vi "ATSpectrograph_getEvent_reportedFilterPosition.vi"(8 "error in (no error)":errorcluster, 11 "logevent_reportedFilterPosition_Ctl":T1) -> (0 "error out":errorcluster, 2 "function return":i32, 3 "logevent_reportedFilterPosition_Ctl out":T1)   [LabVIEW 2016, in "SALLV_ATSpectrograph.lvlib"]
doc: "int ATSpectrograph_shm_getEvent_reportedFilterPositionLV(ATSpectrograph_logevent_reportedFilterPositionLV *logevent_reportedFilterPosition_Ctl );"
uses:
  SALLV_ATSpectrograph.lvlib
  DataTypes/logevent_reportedFilterPosition.ctl
  SALLV_ATSpectrograph.so
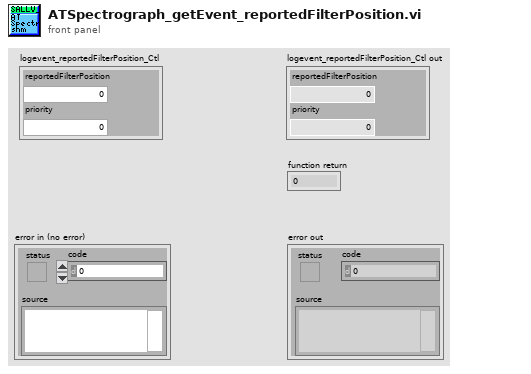
[diagram p1: front panel]
types:
  T1 = typedef "SALLV_ATSpectrograph.lvlib/logevent_reportedFilterPosition.ctl" = cluster{"reportedFilterPosition":i32, "priority":i32}
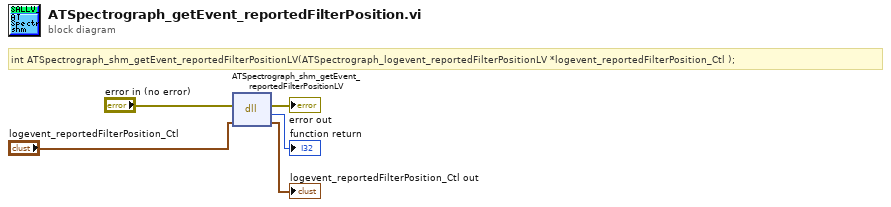
[diagram p0: block diagram]
diagram:
  # "int ATSpectrograph_shm_getEvent_reportedFilterPositionLV(ATSpectrograph_logevent_reportedFilterPositionLV *logevent_reportedFilterPosition_Ctl );"
  n1 = dll-call lib="home/harini/tcs/SALLV_ATSpectrograph/SALLV_ATSpectrograph.*" fn="ATSpectrograph_shm_getEvent_reportedFilterPositionLV"(error in="error in (no error)", "logevent_reportedFilterPosition_Ctl"="logevent_reportedFilterPosition_Ctl") -> (error out=→"error out":errorcluster, →"function return":i32, "logevent_reportedFilterPosition_Ctl"=→"logevent_reportedFilterPosition_Ctl out":T1)  [unwired: 2 in, 1 out]
